vi "encoder.vi"(7 "encoder":cluster{"encoder PPR":dbl, "gear ratio":dbl}, 8 "error in":errorcluster, 9 "encoder reset":bool, 10 "motor  ?":enum16{"M1", "M2", "M3", "M4"}(ring), 11 "FPGA VI Reference":refnum<k20>) -> (0 "error out":errorcluster, 1 "Motor.encoder":dbl, 3 "FPGA VI Reference Out":refnum<k20>)   [LabVIEW 2019, in "my FPGA lib.lvlib" / "motor.lvclass"]
uses:
  motor.lvclass
  <vilib>/Utility/error.llb/Error Cluster From Error Code.vi
  <vilib>/rvi/errors/niLvFpgaAdjustHostInterfaceError.vi
  <vilib>/rvi/interface/nirviReadWriteControl/nirviReadWriteControl.xnode
  NiFpgaLv.dll
  <vilib>/rvi/interface/Simulation/niFpgaSimulationCallBeginRW.vi
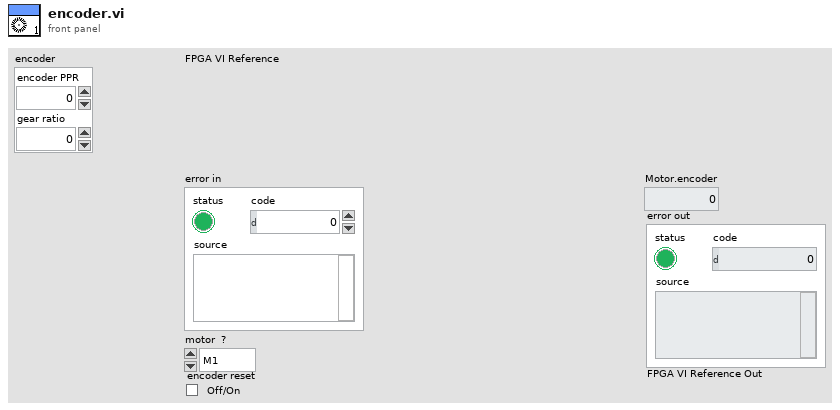
[diagram p1: front panel]
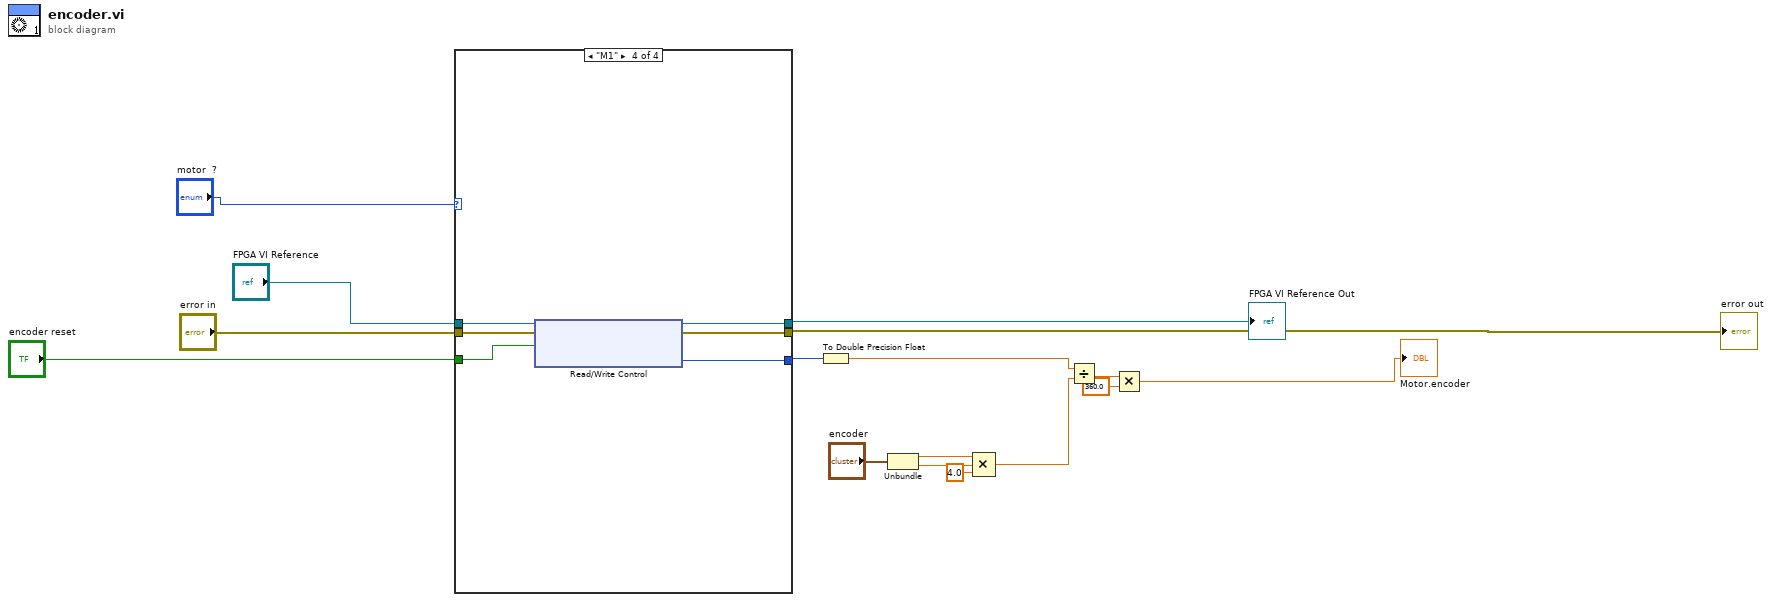
[diagram p0: block diagram]
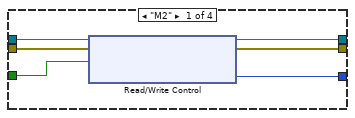
[diagram p2: hidden frame]
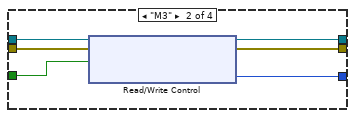
[diagram p3: hidden frame]
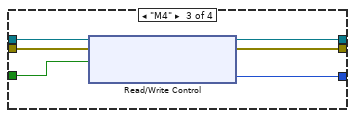
[diagram p4: hidden frame]
diagram:
  n1 = case shown="\"M1\"" "motor  ?" {
    tunnel: "FPGA VI Reference" -> [w22 w28 w34 w40]
    tunnel: "error in" -> [w21 w27 w33 w39]
    tunnel: "encoder reset" -> [w20 w26 w32 w38]
    tunnel: [w19 w25 w31 w37] -> w6
    tunnel: [w18 w24 w30 w36] -> w12
    tunnel: [w17 w23 w29 w35] -> w11
    frame "M2" {
      n2 = xnode "Read/Write Control"("FPGA VI Reference In"=w22, "error in"=w21, "Motor2.encoder_Reset"=w20) -> ("FPGA VI Reference Out"=w17:refnum<k20>, "error out"=w18:errorcluster, "Motor2.encoder"=w19:i32)
    }
    frame "M3" {
      n3 = xnode "Read/Write Control"("FPGA VI Reference In"=w28, "error in"=w27, "Motor3.encoder_Reset"=w26) -> ("FPGA VI Reference Out"=w23:refnum<k20>, "error out"=w24:errorcluster, "Motor3.encoder"=w25:i32)
    }
    frame "M4" {
      n4 = xnode "Read/Write Control"("FPGA VI Reference In"=w34, "error in"=w33, "Motor4.encoder_Reset"=w32) -> ("FPGA VI Reference Out"=w29:refnum<k20>, "error out"=w30:errorcluster, "Motor4.encoder"=w31:i32)
    }
    frame "M1" {
      n5 = xnode "Read/Write Control"("FPGA VI Reference In"=w40, "error in"=w39, "Motor1.encoder_Reset"=w38) -> ("FPGA VI Reference Out"=w35:refnum<k20>, "error out"=w36:errorcluster, "Motor1.encoder"=w37:i32)
    }
  }
  "error out" <- w12
  "FPGA VI Reference Out" <- w11
  n6 = To Double Precision Float(number=w6) -> (double precision float=w5:dbl)
  n7 = Unbundle("encoder") -> ("encoder PPR"=w9:dbl, "gear ratio"=w8:dbl)
  n8 = Compound Arithmetic op=MULTIPLY(w9, w8, 4.0 ("value")) -> (w4:dbl)
  n9 = Divide(x=w5, y=w4) -> (x/y=w3:dbl)
  n10 = Multiply(x=w3, y=360.0) -> (x*y=→"Motor.encoder":dbl)
